vi "write TBM configuration.vi"(8 "error in":errorcluster, 10 "configuration":refnum<class "TBM configuration.lvclass">, 11 "PC in":refnum<class "PLTarget PC.lvclass">) -> (0 "error out":errorcluster, 3 "PC out":refnum<class "PLTarget PC.lvclass">)   [LabVIEW 2013, in "PLTarget PC.lvclass"]
uses:
  PLTarget PC.lvclass
  <vilib>/NI/Tag Bus Module Framework/root configuration/TBM configuration.lvclass
  Framework Configuration Classes/target configuration/PL_Target Configuration.lvclass
  PLTarget PC.lvclass/PLTarget PC.ctl
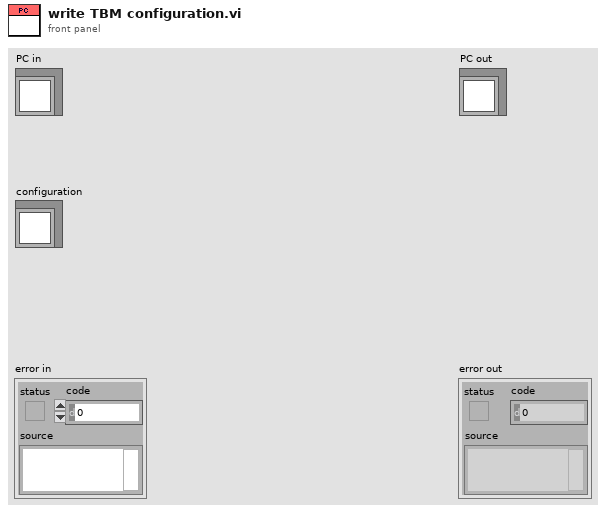
[diagram p1: front panel]
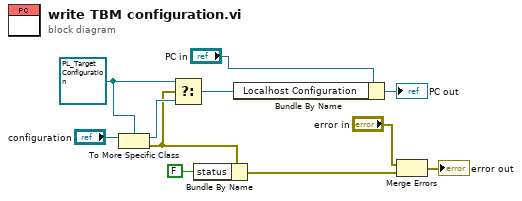
[diagram p0: block diagram]
diagram:
  w4 = refnum<class "PL_Target Configuration.lvclass"> refnum ("Local Target Configuration")
  n1 = To More Specific Class(target class=w4, reference="configuration") -> (specific class reference=w9:refnum<class "PL_Target Configuration.lvclass">, error out=w8:errorcluster)  [unwired: 1 in]
  n2 = Select(t=w4, s=w8, f=w9) -> (s? t:f=w3:refnum<class "PL_Target Configuration.lvclass">)
  n3 = Bundle By Name(cluster=w8, "status"=FALSE) -> (w6:errorcluster)
  n4 = Bundle By Name(cluster="PC in", "Localhost Configuration"=w3) -> (→"PC out":refnum<class "PLTarget PC.lvclass">)
  n5 = Merge Errors("error in", w6) -> (→"error out":errorcluster)
